vi "PID_feedback.vi"(4 "Reset PID and integrator Flag":bool, 5 "currentTensions":dbl[](array[numeric]), 6 "dt (s)":dbl=-1.0 format="%.3f", 9 "desiredTensions":dbl[](array[numeric]), 10 "feedforwardCurrentsIn":dbl[](array[numeric]), 11 "Constants LL":T1) -> (1 "pidCurrentsOut":dbl[](array[numeric]))   [LabVIEW 2024]
uses:
  typeDef/constants_LL.ctl
  <vilib>/addons/control/pid/pid.llb/PID Advanced (DBL Array).vi
  <vilib>/addons/control/pid/pid.llb/PID Parameter Manager (DBL Array).vi
  <vilib>/addons/control/pid/pid.llb/PID Derivative Action Buffered (DBL Array).vi
  <vilib>/addons/control/pid/pid.llb/PID Get Advanced Error (DBL Array).vi
  <vilib>/addons/control/pid/pid.llb/PID Integral Action Buffered (DBL Array).vi
  <vilib>/addons/control/pid/pid.llb/PID Resize 1D Array.vi
  <vilib>/addons/control/pid/pid.llb/PID Get Advanced Error (DBL).vi
  <vilib>/addons/control/pid/NI_PID_pid.lvlib
panel:
  in  "ScalerMin":dbl=1.0
  in  "ScalerRangeMaxTensionInNewtons":dbl=150.0
  in  "ScalerRangeMinTensionInNewtons":dbl=15.0
  in  "ScalerMax":dbl=3.0
  in  "MinimumForOutputUpperBound":dbl=1000.0
  in  "DesiredMinMotorCurrentLimitInMilliAmps":dbl=-1000.0
  in  "PID output range":cluster{"output high":dbl, "output low":dbl}={"output high"=100.0, "output low"=-100.0} {"output low" format="%.2f"; "output high" format="%.2f"}
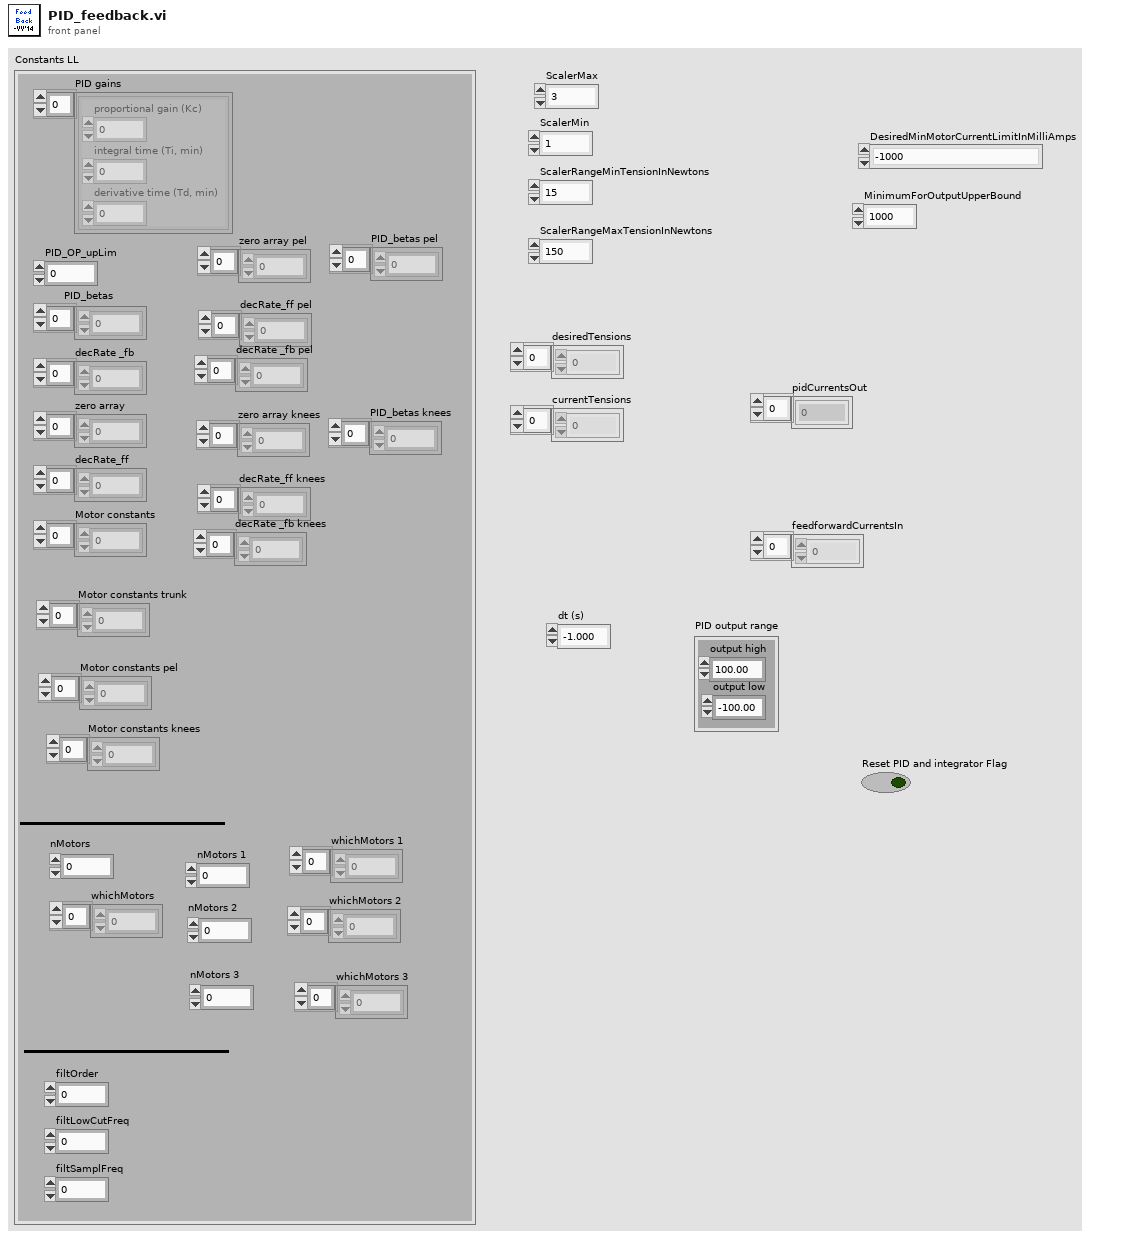
[diagram p1: front panel]
types:
  T1 = typedef "constants_LL.ctl" = cluster{"zero array":dbl[], "decRate_ff":dbl[], "Motor constants":dbl[], "PID gains":cluster{"proportional gain (Kc)":dbl, "integral time (Ti, min)":dbl, "derivative time (Td, min)":dbl}[], "decRate _fb":dbl[], "PID_OP_upLim":dbl, "nMotors":i32, "PID_betas":dbl[], "filtOrder":i32, "filtLowCutFreq":dbl, "filtSamplFreq":dbl, "whichMotors":i32[], "nMotors 1":i32, "nMotors 2":i32, "Motor constants pel":dbl[], "Motor constants trunk":dbl[], "whichMotors 1":i32[], "whichMotors 2":i32[], "zero array pel":dbl[], "decRate_ff pel":dbl[], "decRate _fb pel":dbl[], "PID_betas pel":dbl[], "whichMotors 3":i32[], "nMotors 3":i32, "Motor constants knees":dbl[], "zero array knees":dbl[], "decRate_ff knees":dbl[], "decRate _fb knees":dbl[], "PID_betas knees":dbl[]}
  T2 = cluster{"proportional gain (Kc)":dbl, "integral time (Ti, min)":dbl, "derivative time (Td, min)":dbl}[]
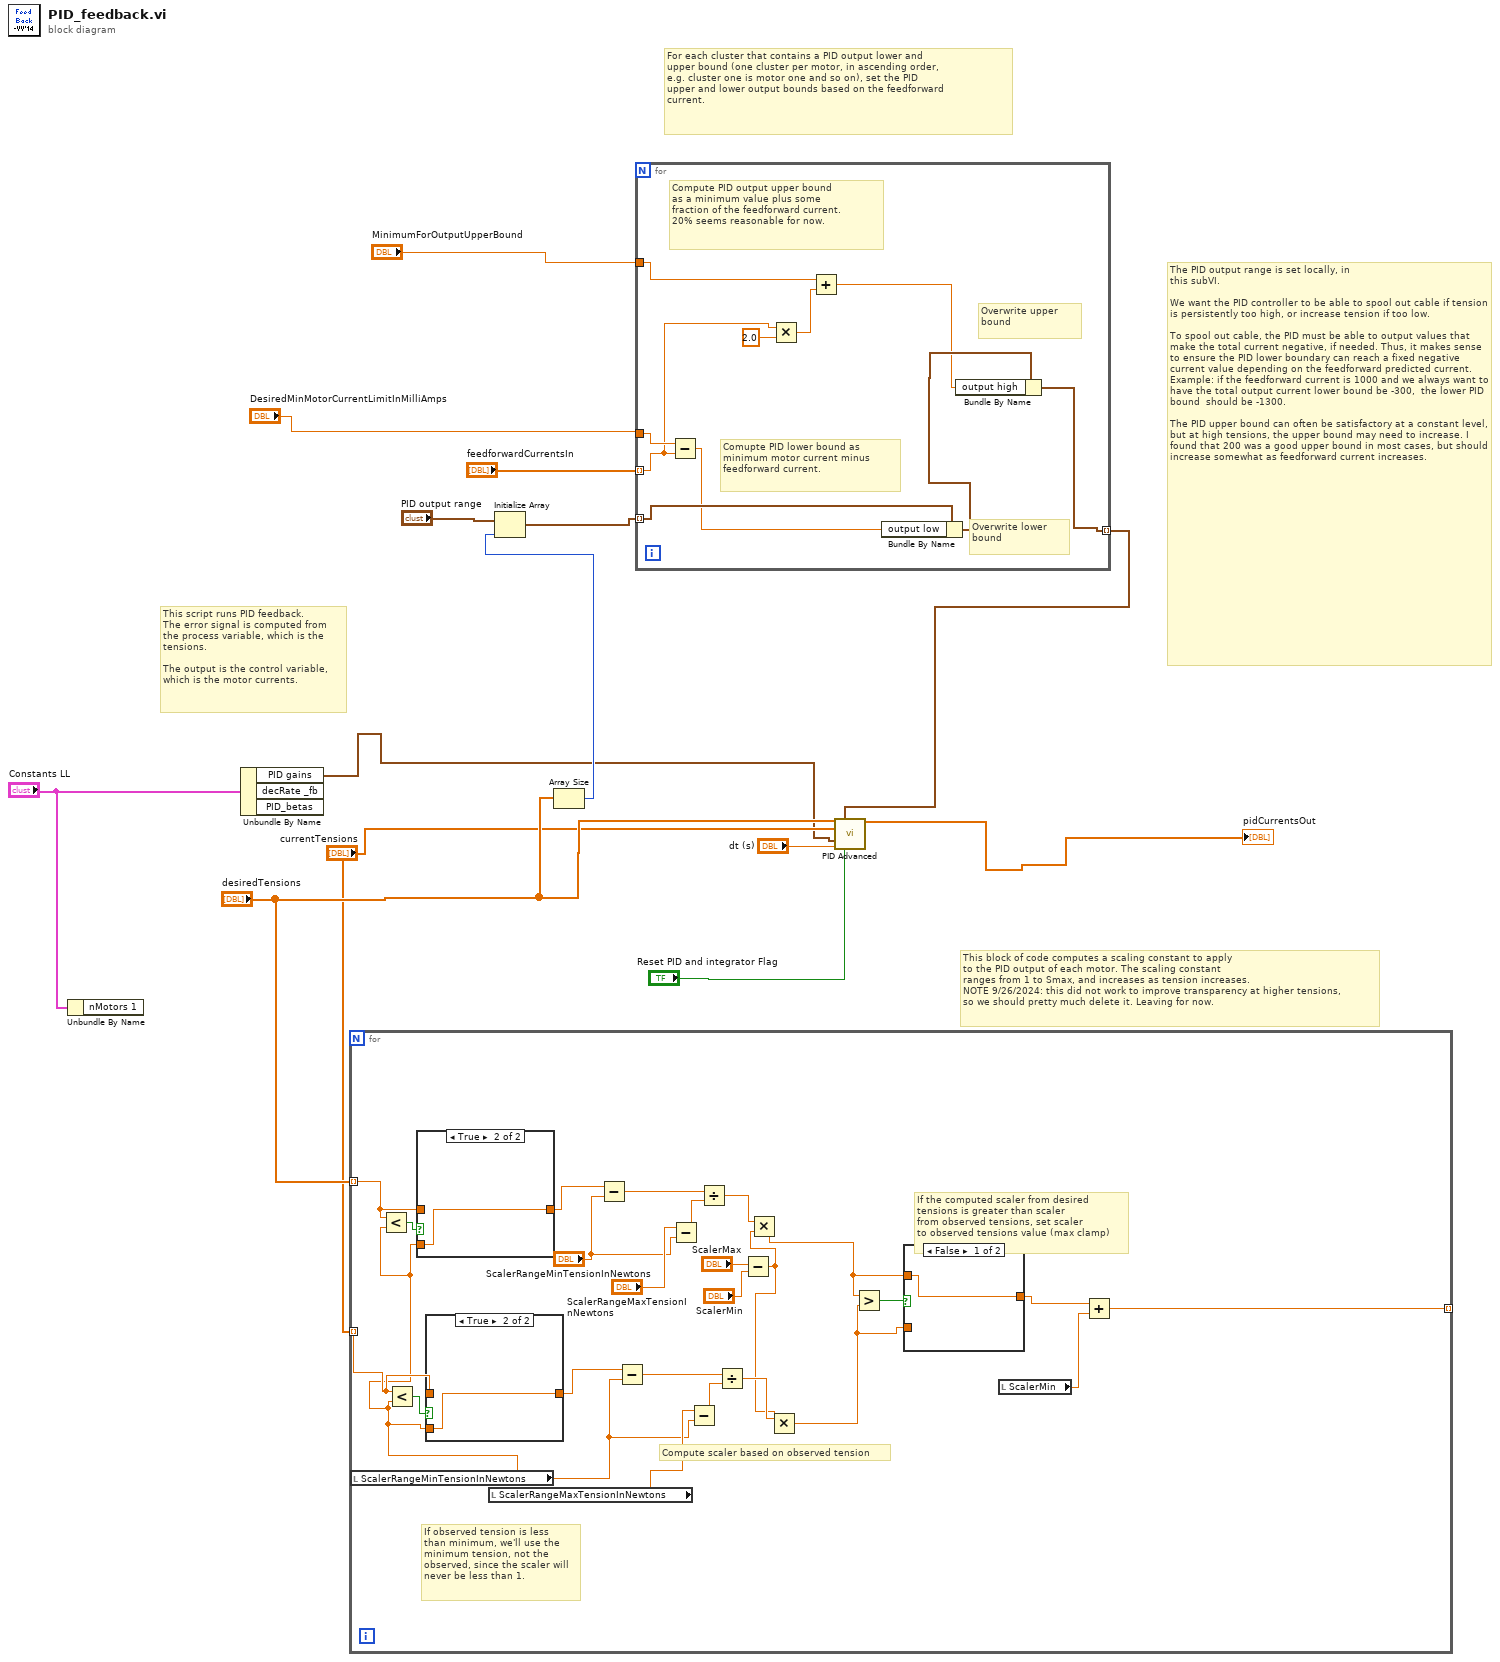
[diagram p0: block diagram]
diagram:
  # "This block of code computes a scaling constant to apply\nto the PID output of each motor. The scaling constant\nranges from 1 to Smax, and increases as tension increases.\nNOTE 9/26/2024: this did not work to improve transparency at higher tensions, \nso we should pretty much delete it. Leaving for now."
  # "For each cluster that contains a PID output lower and \nupper bound (one cluster per motor, in ascending order, \ne.g. cluster one is motor one and so on), set the PID \nupper and lower output bounds based on the feedforward\ncurrent."
  # "The PID output range is set locally, in\nthis subVI.\n\nWe want the PID controller to be able to spool out cable if tension is persistently too high, or increase tension if too low.\n\nTo spool out cable, the PID must be able to output values that make the total current negative, if needed. Thus, it makes sense to ensure the PID lower boundary can reach a fixed negative current value depending on the feedforward predicted current. Example: if the feedforward current is 1000 and we always want to have the total output current lower bound be -300,  the lower PID bound  should be -1300.\n\nThe PID upper bound can often be satisfactory at a constant level, but at high tensions, the upper bound may need to increase. I found that 200 was a good upper bound in most cases, but should increase somewhat as feedforward current increases."
  # "This script runs PID feedback. \nThe error signal is computed from \nthe process variable, which is the \ntensions.\n\nThe output is the control variable, \nwhich is the motor currents."
  n1 = Unbundle By Name("Constants LL") -> ()  [unwired: 1 out]
  n2 = Unbundle By Name("Constants LL") -> ("PID gains"=w2:T2)  [unwired: 2 out]
  n3 = for {
    tunnel: "desiredTensions" -> [w19] mode=indexing
    tunnel: "currentTensions" -> [w26] mode=indexing
    tunnel: [w15] -> _ mode=indexing
    # "If observed tension is less \nthan minimum, we'll use the \nminimum tension, not the \nobserved, since the scaler will\nnever be less than 1."
    # "Compute scaler based on observed tension"
    # "If the computed scaler from desired \ntensions is greater than scaler \nfrom observed tensions, set scaler\nto observed tensions value (max clamp)"
    n4 = local read "ScalerRangeMinTensionInNewtons"() -> (w18:dbl)
    n5 = Less?(x=w19, y=w18) -> (x < y?=w16:bool)
    n6 = Less?(x=w26, y=w18) -> (x < y?=w28:bool)
    n7 = case shown="True" w16 {
      tunnel: w18 -> [_ w41]
      tunnel: [w40 w41] -> w17
      tunnel: w19 -> [w40 _]
      frame False {
      }
      frame True {
      }
    }
    n8 = case shown="True" w28 {
      tunnel: w18 -> [_ w43]
      tunnel: [w42 w43] -> w25
      tunnel: w26 -> [w42 _]
      frame False {
      }
      frame True {
      }
    }
    n9 = local read "ScalerRangeMaxTensionInNewtons"() -> (w27:dbl)
    n10 = Subtract(x=w17, y="ScalerRangeMinTensionInNewtons") -> (x-y=w37:dbl)
    n11 = Subtract(x=w25, y=w18) -> (x-y=w34:dbl)
    n12 = Subtract(x="ScalerRangeMaxTensionInNewtons", y="ScalerRangeMinTensionInNewtons") -> (x-y=w36:dbl)
    n13 = Subtract(x=w27, y=w18) -> (x-y=w33:dbl)
    n14 = Divide(x=w37, y=w36) -> (x/y=w35:dbl)
    n15 = Divide(x=w34, y=w33) -> (x/y=w32:dbl)
    n16 = Subtract(x="ScalerMax", y="ScalerMin") -> (x-y=w22:dbl)
    n17 = Multiply(x=w35, y=w22) -> (x*y=w29:dbl)
    n18 = Multiply(x=w32, y=w22) -> (x*y=w30:dbl)
    n19 = Greater?(x=w29, y=w30) -> (0:w31:bool)
    n20 = case shown="False" w31 {
      tunnel: w30 -> [_ w45]
      tunnel: w29 -> [w44 _]
      tunnel: [w44 w45] -> w20
      frame False {
      }
      frame True {
      }
    }
    n21 = local read "ScalerMin"() -> (w21:dbl)
    n22 = Add(x=w20, y=w21) -> (x+y=w15:dbl)
  }
  n23 = Array Size(array="desiredTensions") -> (size(s)=w10:i32)
  n24 = Initialize Array("PID output range", w10) -> (w7:cluster{"output high":dbl, "output low":dbl}[])
  n25 = for {
    tunnel: "feedforwardCurrentsIn" -> [w51] mode=indexing
    tunnel: "DesiredMinMotorCurrentLimitInMilliAmps" -> [w55]
    tunnel: w7 -> [w54] mode=indexing
    tunnel: [w46] -> w6 mode=indexing
    tunnel: "MinimumForOutputUpperBound" -> [w50]
    # "Overwrite upper \nbound"
    # "Overwrite lower \nbound"
    # "Compute PID output upper bound \nas a minimum value plus some \nfraction of the feedforward current. \n20% seems reasonable for now."
    # "Comupte PID lower bound as \nminimum motor current minus\nfeedforward current."
    n26 = Subtract(x=w55, y=w51) -> (x-y=w53:dbl)
    n27 = Multiply(x=w51, y=2.0) -> (x*y=w49:dbl)
    n28 = Add(x=w50, y=w49) -> (x+y=w47:dbl)
    n29 = Bundle By Name(cluster=w54, "output low"=w53) -> (w48:cluster{"output high":dbl, "output low":dbl})
    n30 = Bundle By Name(cluster=w48, "output high"=w47) -> (w46:cluster{"output high":dbl, "output low":dbl})
  }
  n31 = call-poly <vilib>:"PID Advanced.vi"("setpoint"="desiredTensions", "output range"=w6, "process variable"="currentTensions", "PID gains"=w2, "dt (s)"="dt (s)", "reinitialize? (F)"="Reset PID and integrator Flag") -> ("output"=→"pidCurrentsOut":dbl[])  [unwired: 8 in, 1 out]
